vi "Read GoToBallPlacementPositionTactic.vi"(8 "error in (no error)":errorcluster, 11 "Tacticbook in":refnum<class "Tacticbook.lvclass">) -> (0 "error out":errorcluster, 2 "GoToBallPlacementPositionTactic":refnum<class "GoToBallPlacementPositionTactic.lvclass">, 3 "Tacticbook out":refnum<class "Tacticbook.lvclass">)   [LabVIEW 2021, in "Tacticbook.lvclass"]
uses:
  Tacticbook.lvclass
  GoToBallPlacementPositionTactic_class/GoToBallPlacementPositionTactic.lvclass
  Tacticbook.lvclass/Tacticbook.ctl
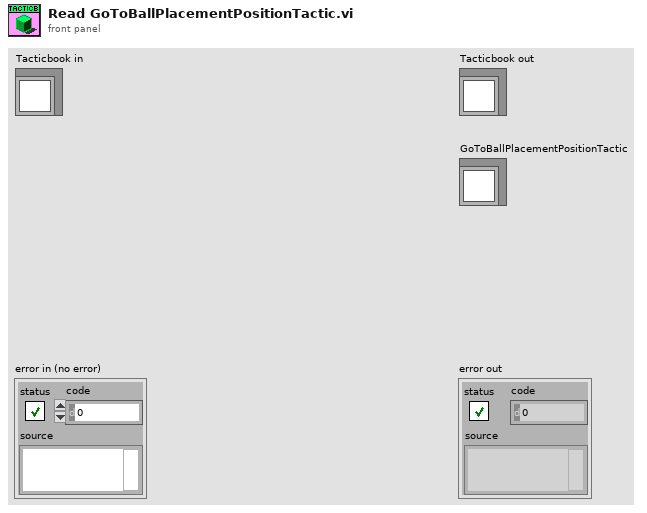
[diagram p1: front panel]
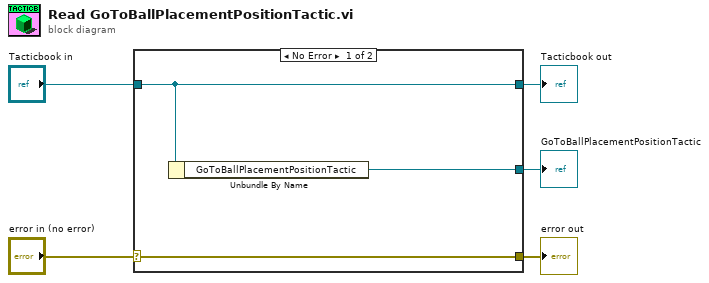
[diagram p0: block diagram]
diagram:
  n1 = case shown="No Error" "error in (no error)" {
    selector: "error in (no error)" -> [w8 w9]
    tunnel: [w8 w9] -> w4
    tunnel: [w7 w10] -> w2
    tunnel: "Tacticbook in" -> [w7 w10]
    tunnel: [w6 _] -> w1
    frame No Error {
      n2 = Unbundle By Name(w7) -> ("GoToBallPlacementPositionTactic"=w6:refnum<class "GoToBallPlacementPositionTactic.lvclass">)
    }
    frame Error {
    }
  }
  "error out" <- w4
  "Tacticbook out" <- w2
  "GoToBallPlacementPositionTactic" <- w1
